vi "InitSupervisorCluster.vi"(8 "error in (no error)":errorcluster, 11 "ClusterIn in":T1={"Admin"={"Lvl"=enum."Admin", "Pwd"=""}, "RTConfig"={"Arm"=FALSE, "Number"=0.0, "String"=""}, "SMS"={"Enbl?"=FALSE, "Addr"=[]}, "FPGA"={"Target"=enum."1", "Channel"=enum."1", "Ref1"=refnum, "Ref2"=refnum}, "Config"={"UsrCfg"={"Paths"={"CfgFile"=path "", "LogFolder"=path "", "LogFile"=path "", "NAS path"=path "", "ThreshFile"=path "", "RedunFolder"=path ""}, "SampleRate"=0.0}, "FP_User"={"#NoiseSums"=0, "Max_df"=0, "AvgAvg"=FALSE, "#Avg"=0, "AutoCenter"=FALSE, "Inclin"={"Vmin"=0.0, "Vmax"=0.0, "Angle_min"=0.0, "Angle_max"=0.0, "Offset"=0.0, "Pos_Neg"=FALSE}, "1"={"Cal_"={"Fine"=0.0, "Coarse_"=0.0}, "Beac"={"Fine"=0.0, "Coarse_"=0.0}, "Scale"={"Step4"=0.0, "Step5"=0.0, "Step6"=0.0, "Step7"=0.0}, "Offset"=0.0, "Scale_Noise"=0.0, "Scale_Step1"=0.0, "Scale_In_RT"=0.0, "ScaleMeas"=0.0, "FreqsToRemove"=[], "Width"=[], "ScaleMeasEnum"=enum."1", "FilterEnab"=enum."None"}, "2"={"Cal_"={"Fine"=0.0, "Coarse_"=0.0}, "Beac"={"Fine"=0.0, "Coarse_"=0.0}, "Scale"={"Step4"=0.0, "Step5"=0.0, "Step6"=0.0, "Step7"=0.0}, "Offset"=0.0, "Scale_Noise"=0.0, "Scale_Step1"=0.0, "Scale_In_RT"=0.0, "ScaleMeas"=0.0, "FreqsToRemove"=[], "Width"=[], "ScaleMeasEnum"=enum."1", "FilterEnab"=enum."None"}, "3"={"Cal_"={"Fine"=0.0, "Coarse_"=0.0}, "Beac"={"Fine"=0.0, "Coarse_"=0.0}, "Scale"={"Step4"=0.0, "Step5"=0.0, "Step6"=0.0, "Step7"=0.0}, "Offset"=0.0, "Scale_Noise"=0.0, "Scale_Step1"=0.0, "Scale_In_RT"=0.0, "ScaleMeas"=0.0, "FreqsToRemove"=[], "Width"=[], "ScaleMeasEnum"=enum."1", "FilterEnab"=enum."None"}, "4"={"Cal_"={"Fine"=0.0, "Coarse_"=0.0}, "Beac"={"Fine"=0.0, "Coarse_"=0.0}, "Scale"={"Step4"=0.0, "Step5"=0.0, "Step6"=0.0, "Step7"=0.0}, "Offset"=0.0, "Scale_Noise"=0.0, "Scale_Step1"=0.0, "Scale_In_RT"=0.0, "ScaleMeas"=0.0, "FreqsToRemove"=[], "Width"=[], "ScaleMeasEnum"=enum."1", "FilterEnab"=enum."None"}, "Target to Probe"=enum."1", "SNR_Thresh"=0.0, "Paths"={"CfgFile"=path "", "LogFolder"=path "", "LogFile"=path "", "NAS path"=path "", "ThreshFile"=path "", "RedunFolder"=path ""}, "Connex_Location"="", "SimulateFPGA"=FALSE, "Deadband"=0.0}}, "Stat"={"SysState"=enum."Init", "TrackRate"=FALSE, "AutoCentr"=FALSE}, "Alarm"={"TC13"={"Enbl"=FALSE, "ErrsAndWarns"={0.0, 5.663716814159292, 7.168141592920354, 8.584070796460177}}, "AI1"={"Enbl"=FALSE, "ErrsAndWarns"={0.0, 5.663716814159292, 7.168141592920354, 8.584070796460177}}, "AI2"={"Enbl"=FALSE, "ErrsAndWarns"={0.0, 5.663716814159292, 7.168141592920354, 8.584070796460177}}, "AI3"={"Enbl"=FALSE, "ErrsAndWarns"={0.0, 5.663716814159292, 7.168141592920354, 8.584070796460177}}, "AI4"={"Enbl"=FALSE, "ErrsAndWarns"={0.0, 5.663716814159292, 7.168141592920354, 8.584070796460177}}, "AI5"={"Enbl"=FALSE, "ErrsAndWarns"={0.0, 5.663716814159292, 7.168141592920354, 8.584070796460177}}, "AI6"={"Enbl"=FALSE, "ErrsAndWarns"={0.0, 5.663716814159292, 7.168141592920354, 8.584070796460177}}, "AI18"={"Enbl"=FALSE, "ErrsAndWarns"={0.0, 5.663716814159292, 7.168141592920354, 8.584070796460177}}, "AI19"={"Enbl"=FALSE, "ErrsAndWarns"={0.0, 5.663716814159292, 7.168141592920354, 8.584070796460177}}, "TE1"={"Enbl"=FALSE, "ErrsAndWarns"={0.0, 5.663716814159292, 7.168141592920354, 8.584070796460177}}, "TE2"={"Enbl"=TRUE, "ErrsAndWarns"={0.0, 5.663716814159292, 7.168141592920354, 8.584070796460177}}, "TE3"={"Enbl"=FALSE, "ErrsAndWarns"={0.0, 5.663716814159292, 7.168141592920354, 8.584070796460177}}, "ADAM1"={"Enbl"=FALSE, "ErrsAndWarns"={0.0, 5.663716814159292, 7.168141592920354, 8.584070796460177}}, "ADAM2"={"Enbl"=FALSE, "ErrsAndWarns"={0.0, 5.663716814159292, 7.168141592920354, 8.584070796460177}}, "ADAM3"={"Enbl"=FALSE, "ErrsAndWarns"={0.0, 5.663716814159292, 7.168141592920354, 8.584070796460177}}, "ADAM4"={"Enbl"=FALSE, "ErrsAndWarns"={0.0, 5.663716814159292, 7.168141592920354, 8.584070796460177}}, "72CoBeacFreq"={"Enbl"=FALSE, "ErrsAndWarns"={0.0, 5.663716814159292, 7.168141592920354, 8.584070796460177}}, "72CoCalFreq"={"Enbl"=FALSE, "ErrsAndWarns"={0.0, 5.663716814159292, 7.168141592920354, 8.584070796460177}}, "84CoBeacFreq"={"Enbl"=FALSE, "ErrsAndWarns"={0.0, 5.663716814159292, 7.168141592920354, 8.584070796460177}}, "84CoCalFreq"={"Enbl"=FALSE, "ErrsAndWarns"={0.0, 5.663716814159292, 7.168141592920354, 8.584070796460177}}, "72Co_CalTonePwr"={"Enbl"=FALSE, "ErrsAndWarns"={0.0, 5.663716814159292, 7.168141592920354, 8.584070796460177}}, "72X_CalTonePwr"={"Enbl"=FALSE, "ErrsAndWarns"={0.0, 5.663716814159292, 7.168141592920354, 8.584070796460177}}, "84Co_CalTonePwr"={"Enbl"=FALSE, "ErrsAndWarns"={0.0, 5.663716814159292, 7.168141592920354, 8.584070796460177}}, "84X_CalTonePwr"={"Enbl"=FALSE, "ErrsAndWarns"={0.0, 5.663716814159292, 7.168141592920354, 8.584070796460177}}}} {"Alarm"."84X_CalTonePwr"."ErrsAndWarns" scale=-120.0..-45.0; "Alarm"."72X_CalTonePwr"."ErrsAndWarns" scale=-120.0..-45.0; "Alarm"."84Co_CalTonePwr"."ErrsAndWarns" scale=-120.0..-45.0; "Alarm"."72Co_CalTonePwr"."ErrsAndWarns" scale=-120.0..-45.0; "Alarm"."84CoCalFreq"."ErrsAndWarns" scale=24.9..25.1; "Alarm"."84CoBeacFreq"."ErrsAndWarns" scale=25.5..27.0; "Alarm"."72CoCalFreq"."ErrsAndWarns" scale=24.9..25.1; "Alarm"."72CoBeacFreq"."ErrsAndWarns" scale=25.5..27.0; "Alarm"."ADAM4"."ErrsAndWarns" scale=30.0..52.0; "Alarm"."ADAM3"."ErrsAndWarns" scale=30.0..52.0; "Alarm"."ADAM2"."ErrsAndWarns" scale=30.0..52.0; "Alarm"."ADAM1"."ErrsAndWarns" scale=30.0..52.0; "Alarm"."TE3"."ErrsAndWarns" scale=30.0..52.0; "Alarm"."TE2"."ErrsAndWarns" scale=30.0..52.0; "Alarm"."TE1"."ErrsAndWarns" scale=20.0..52.0; "Alarm"."AI19"."ErrsAndWarns" scale=0.0..60.0; "Alarm"."AI18"."ErrsAndWarns" scale=-10.0..10.0; "Alarm"."AI6"."ErrsAndWarns" scale=0.0..35.0; "Alarm"."AI5"."ErrsAndWarns" scale=0.0..20.0; "Alarm"."AI4"."ErrsAndWarns" scale=0.0..15.0; "Alarm"."AI3"."ErrsAndWarns" scale=0.0..10.0; "Alarm"."AI2"."ErrsAndWarns" scale=0.0..10.0; "Alarm"."TC13"."ErrsAndWarns" scale=-10.0..40.0; "Config"."FP_User"."Deadband" format="%#.0f"}) -> (0 "error out":errorcluster, 3 "ClusterIn out":T1={"Admin"={"Lvl"=enum."Admin", "Pwd"=""}, "RTConfig"={"Arm"=FALSE, "Number"=0.0, "String"=""}, "SMS"={"Enbl?"=FALSE, "Addr"=[]}, "FPGA"={"Target"=enum."1", "Channel"=enum."1", "Ref1"=refnum, "Ref2"=refnum}, "Config"={"UsrCfg"={"Paths"={"CfgFile"=path "", "LogFolder"=path "", "LogFile"=path "", "NAS path"=path "", "ThreshFile"=path "", "RedunFolder"=path ""}, "SampleRate"=0.0}, "FP_User"={"#NoiseSums"=0, "Max_df"=0, "AvgAvg"=FALSE, "#Avg"=0, "AutoCenter"=FALSE, "Inclin"={"Vmin"=0.0, "Vmax"=0.0, "Angle_min"=0.0, "Angle_max"=0.0, "Offset"=0.0, "Pos_Neg"=FALSE}, "1"={"Cal_"={"Fine"=0.0, "Coarse_"=0.0}, "Beac"={"Fine"=0.0, "Coarse_"=0.0}, "Scale"={"Step4"=0.0, "Step5"=0.0, "Step6"=0.0, "Step7"=0.0}, "Offset"=0.0, "Scale_Noise"=0.0, "Scale_Step1"=0.0, "Scale_In_RT"=0.0, "ScaleMeas"=0.0, "FreqsToRemove"=[], "Width"=[], "ScaleMeasEnum"=enum."1", "FilterEnab"=enum."None"}, "2"={"Cal_"={"Fine"=0.0, "Coarse_"=0.0}, "Beac"={"Fine"=0.0, "Coarse_"=0.0}, "Scale"={"Step4"=0.0, "Step5"=0.0, "Step6"=0.0, "Step7"=0.0}, "Offset"=0.0, "Scale_Noise"=0.0, "Scale_Step1"=0.0, "Scale_In_RT"=0.0, "ScaleMeas"=0.0, "FreqsToRemove"=[], "Width"=[], "ScaleMeasEnum"=enum."1", "FilterEnab"=enum."None"}, "3"={"Cal_"={"Fine"=0.0, "Coarse_"=0.0}, "Beac"={"Fine"=0.0, "Coarse_"=0.0}, "Scale"={"Step4"=0.0, "Step5"=0.0, "Step6"=0.0, "Step7"=0.0}, "Offset"=0.0, "Scale_Noise"=0.0, "Scale_Step1"=0.0, "Scale_In_RT"=0.0, "ScaleMeas"=0.0, "FreqsToRemove"=[], "Width"=[], "ScaleMeasEnum"=enum."1", "FilterEnab"=enum."None"}, "4"={"Cal_"={"Fine"=0.0, "Coarse_"=0.0}, "Beac"={"Fine"=0.0, "Coarse_"=0.0}, "Scale"={"Step4"=0.0, "Step5"=0.0, "Step6"=0.0, "Step7"=0.0}, "Offset"=0.0, "Scale_Noise"=0.0, "Scale_Step1"=0.0, "Scale_In_RT"=0.0, "ScaleMeas"=0.0, "FreqsToRemove"=[], "Width"=[], "ScaleMeasEnum"=enum."1", "FilterEnab"=enum."None"}, "Target to Probe"=enum."1", "SNR_Thresh"=0.0, "Paths"={"CfgFile"=path "", "LogFolder"=path "", "LogFile"=path "", "NAS path"=path "", "ThreshFile"=path "", "RedunFolder"=path ""}, "Connex_Location"="", "SimulateFPGA"=FALSE, "Deadband"=0.0}}, "Stat"={"SysState"=enum."Init", "TrackRate"=FALSE, "AutoCentr"=FALSE}, "Alarm"={"TC13"={"Enbl"=FALSE, "ErrsAndWarns"={0.0, 5.663716814159292, 7.168141592920354, 8.584070796460177}}, "AI1"={"Enbl"=FALSE, "ErrsAndWarns"={0.0, 5.663716814159292, 7.168141592920354, 8.584070796460177}}, "AI2"={"Enbl"=FALSE, "ErrsAndWarns"={0.0, 5.663716814159292, 7.168141592920354, 8.584070796460177}}, "AI3"={"Enbl"=FALSE, "ErrsAndWarns"={0.0, 5.663716814159292, 7.168141592920354, 8.584070796460177}}, "AI4"={"Enbl"=FALSE, "ErrsAndWarns"={0.0, 5.663716814159292, 7.168141592920354, 8.584070796460177}}, "AI5"={"Enbl"=FALSE, "ErrsAndWarns"={0.0, 5.663716814159292, 7.168141592920354, 8.584070796460177}}, "AI6"={"Enbl"=FALSE, "ErrsAndWarns"={0.0, 5.663716814159292, 7.168141592920354, 8.584070796460177}}, "AI18"={"Enbl"=FALSE, "ErrsAndWarns"={0.0, 5.663716814159292, 7.168141592920354, 8.584070796460177}}, "AI19"={"Enbl"=FALSE, "ErrsAndWarns"={0.0, 5.663716814159292, 7.168141592920354, 8.584070796460177}}, "TE1"={"Enbl"=FALSE, "ErrsAndWarns"={0.0, 5.663716814159292, 7.168141592920354, 8.584070796460177}}, "TE2"={"Enbl"=TRUE, "ErrsAndWarns"={0.0, 5.663716814159292, 7.168141592920354, 8.584070796460177}}, "TE3"={"Enbl"=FALSE, "ErrsAndWarns"={0.0, 5.663716814159292, 7.168141592920354, 8.584070796460177}}, "ADAM1"={"Enbl"=FALSE, "ErrsAndWarns"={0.0, 5.663716814159292, 7.168141592920354, 8.584070796460177}}, "ADAM2"={"Enbl"=FALSE, "ErrsAndWarns"={0.0, 5.663716814159292, 7.168141592920354, 8.584070796460177}}, "ADAM3"={"Enbl"=FALSE, "ErrsAndWarns"={0.0, 5.663716814159292, 7.168141592920354, 8.584070796460177}}, "ADAM4"={"Enbl"=FALSE, "ErrsAndWarns"={0.0, 5.663716814159292, 7.168141592920354, 8.584070796460177}}, "72CoBeacFreq"={"Enbl"=FALSE, "ErrsAndWarns"={0.0, 5.663716814159292, 7.168141592920354, 8.584070796460177}}, "72CoCalFreq"={"Enbl"=FALSE, "ErrsAndWarns"={0.0, 5.663716814159292, 7.168141592920354, 8.584070796460177}}, "84CoBeacFreq"={"Enbl"=FALSE, "ErrsAndWarns"={0.0, 5.663716814159292, 7.168141592920354, 8.584070796460177}}, "84CoCalFreq"={"Enbl"=FALSE, "ErrsAndWarns"={0.0, 5.663716814159292, 7.168141592920354, 8.584070796460177}}, "72Co_CalTonePwr"={"Enbl"=FALSE, "ErrsAndWarns"={0.0, 5.663716814159292, 7.168141592920354, 8.584070796460177}}, "72X_CalTonePwr"={"Enbl"=FALSE, "ErrsAndWarns"={0.0, 5.663716814159292, 7.168141592920354, 8.584070796460177}}, "84Co_CalTonePwr"={"Enbl"=FALSE, "ErrsAndWarns"={0.0, 5.663716814159292, 7.168141592920354, 8.584070796460177}}, "84X_CalTonePwr"={"Enbl"=FALSE, "ErrsAndWarns"={0.0, 5.663716814159292, 7.168141592920354, 8.584070796460177}}}} {"Alarm"."84X_CalTonePwr"."ErrsAndWarns" scale=-120.0..-45.0; "Alarm"."72X_CalTonePwr"."ErrsAndWarns" scale=-120.0..-45.0; "Alarm"."84Co_CalTonePwr"."ErrsAndWarns" scale=-120.0..-45.0; "Alarm"."72Co_CalTonePwr"."ErrsAndWarns" scale=-120.0..-45.0; "Alarm"."84CoCalFreq"."ErrsAndWarns" scale=24.9..25.1; "Alarm"."84CoBeacFreq"."ErrsAndWarns" scale=25.5..27.0; "Alarm"."72CoCalFreq"."ErrsAndWarns" scale=24.9..25.1; "Alarm"."72CoBeacFreq"."ErrsAndWarns" scale=25.5..27.0; "Alarm"."ADAM4"."ErrsAndWarns" scale=30.0..52.0; "Alarm"."ADAM3"."ErrsAndWarns" scale=30.0..52.0; "Alarm"."ADAM2"."ErrsAndWarns" scale=30.0..52.0; "Alarm"."ADAM1"."ErrsAndWarns" scale=30.0..52.0; "Alarm"."TE3"."ErrsAndWarns" scale=30.0..52.0; "Alarm"."TE2"."ErrsAndWarns" scale=30.0..52.0; "Alarm"."TE1"."ErrsAndWarns" scale=20.0..52.0; "Alarm"."AI19"."ErrsAndWarns" scale=0.0..60.0; "Alarm"."AI18"."ErrsAndWarns" scale=-10.0..10.0; "Alarm"."AI6"."ErrsAndWarns" scale=0.0..35.0; "Alarm"."AI5"."ErrsAndWarns" scale=0.0..20.0; "Alarm"."AI4"."ErrsAndWarns" scale=0.0..15.0; "Alarm"."AI3"."ErrsAndWarns" scale=0.0..10.0; "Alarm"."AI2"."ErrsAndWarns" scale=0.0..10.0; "Alarm"."TC13"."ErrsAndWarns" scale=-10.0..40.0; "Config"."FP_User"."Deadband" format="%#.0f"})   [LabVIEW 2018]
uses:
  Controls/MasterCluster.ctl
  Controls/Clusts/AdminCluster.ctl
  Controls/UserLevelEnum.ctl
  Controls/RT_Config.ctl
  Controls/SMSDataCluster.ctl
  Controls/Clusts/FPGA_Config_Clust.ctl
  Controls/Enums/TargetNumber.ctl
  Controls/Clusts/Config_Clust.ctl
  Controls/Clusts/UserConfig.ctl
  Controls/PathsCluster.ctl
  Controls/Clusts/FrontPanel_UserConfig.ctl
  Controls/Clusts/Inclinometer_User_Cfg.ctl
  Controls/Clusts/FP_UserTargetConfig.ctl
  Controls/Clusts/FreqShift.ctl
  Controls/Clusts/FPGA_Scale.ctl
  Controls/Enums/ScaleMeasure.ctl
  Controls/RadioButtons/FilterEnableRadio.ctl
  Controls/SystemStatusCluster.ctl
  Controls/SystemStateEnum.ctl
  Controls/Clusts/AlarmSettingsClust.ctl
  Controls/Clusts/AlarmThresh_OneChan.ctl
  <vilib>/Utility/sysdir.llb/System Directory Type.ctl
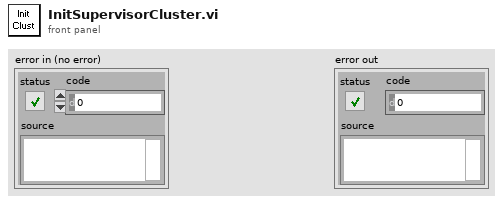
[diagram p1: front panel]
types:
  T1 = typedef "MasterCluster.ctl" = cluster{"Admin":T2, "RTConfig":T4, "SMS":T5, "FPGA":T6, "Config":T8, "Stat":T18, "Alarm":T20}
  T2 = typedef "AdminCluster.ctl" = cluster{"Lvl":T3, "Pwd":string}
  T3 = typedef "UserLevelEnum.ctl" = enum16{"Admin", "Operator"}
  T4 = typedef "RT_Config.ctl" = cluster{"Arm":bool, "Number":dbl, "String":string}
  T5 = typedef "SMSDataCluster.ctl" = cluster{"Enbl?":bool, "Addr":string[]}
  T6 = typedef "FPGA_Config_Clust.ctl" = cluster{"Target":T7, "Channel":T7, "Ref1":refnum<k20>, "Ref2":refnum<k20>}
  T7 = typedef "TargetNumber.ctl" = enum16{"1", "2", "3", "4"}
  T8 = typedef "Config_Clust.ctl" = cluster{"UsrCfg":T9, "FP_User":T11}
  T9 = typedef "UserConfig.ctl" = cluster{"Paths":T10, "SampleRate":dbl}
  T10 = typedef "PathsCluster.ctl" = cluster{"CfgFile":path, "LogFolder":path, "LogFile":path, "NAS path":path, "ThreshFile":path, "RedunFolder":path}
  T11 = typedef "FrontPanel_UserConfig.ctl" = cluster{"#NoiseSums":u32, "Max_df":u32, "AvgAvg":bool, "#Avg":u16, "AutoCenter":bool, "Inclin":T12, "1":T13, "2":T13, "3":T13, "4":T13, "Target to Probe":T7, "SNR_Thresh":dbl, "Paths":T10, "Connex_Location":string, "SimulateFPGA":bool, "Deadband":dbl}
  T12 = typedef "Inclinometer_User_Cfg.ctl" = cluster{"Vmin":dbl, "Vmax":dbl, "Angle_min":dbl, "Angle_max":dbl, "Offset":dbl, "Pos_Neg":bool}
  T13 = typedef "FP_UserTargetConfig.ctl" = cluster{"Cal_":T14, "Beac":T14, "Scale":T15, "Offset":fxp<+/-,16,16>, "Scale_Noise":fxp<+/-,30,30>, "Scale_Step1":fxp<+/-,17,17>, "Scale_In_RT":ext, "ScaleMeas":fxp<+/-,16,1>, "FreqsToRemove":i32[], "Width":i32[], "ScaleMeasEnum":T16, "FilterEnab":T17}
  T14 = typedef "FreqShift.ctl" = cluster{"Fine":dbl, "Coarse_":dbl}
  T15 = typedef "FPGA_Scale.ctl" = cluster{"Step4":fxp<+/-,23,23>, "Step5":fxp<+/-,23,23>, "Step6":fxp<+/-,23,23>, "Step7":fxp<+/-,23,23>}
  T16 = typedef "ScaleMeasure.ctl" = enum16{"1", "10", "50", "42"}
  T17 = typedef "FilterEnableRadio.ctl" = enum32{"None", "Step 1", "Frequency Shift", "Step 4", "Step 5", "Step 6", "Step 7"}
  T18 = typedef "SystemStatusCluster.ctl" = cluster{"SysState":T19, "TrackRate":bool, "AutoCentr":bool}
  T19 = typedef "SystemStateEnum.ctl" = enum16{"Init", "Idle", "Running", "System Fault", "System Error", "Exit"}
  T20 = typedef "AlarmSettingsClust.ctl" = cluster{"TC13":T21, "AI1":T21, "AI2":T21, "AI3":T21, "AI4":T21, "AI5":T21, "AI6":T21, "AI18":T21, "AI19":T21, "TE1":T21, "TE2":T21, "TE3":T21, "ADAM1":T21, "ADAM2":T21, "ADAM3":T21, "ADAM4":T21, "72CoBeacFreq":T21, "72CoCalFreq":T21, "84CoBeacFreq":T21, "84CoCalFreq":T21, "72Co_CalTonePwr":T21, "72X_CalTonePwr":T21, "84Co_CalTonePwr":T21, "84X_CalTonePwr":T21}
  T21 = typedef "AlarmThresh_OneChan.ctl" = cluster{"Enbl":bool, "ErrsAndWarns":cluster{dbl, dbl, dbl, dbl}}
  T22 = typedef "System Directory Type.ctl" = i32
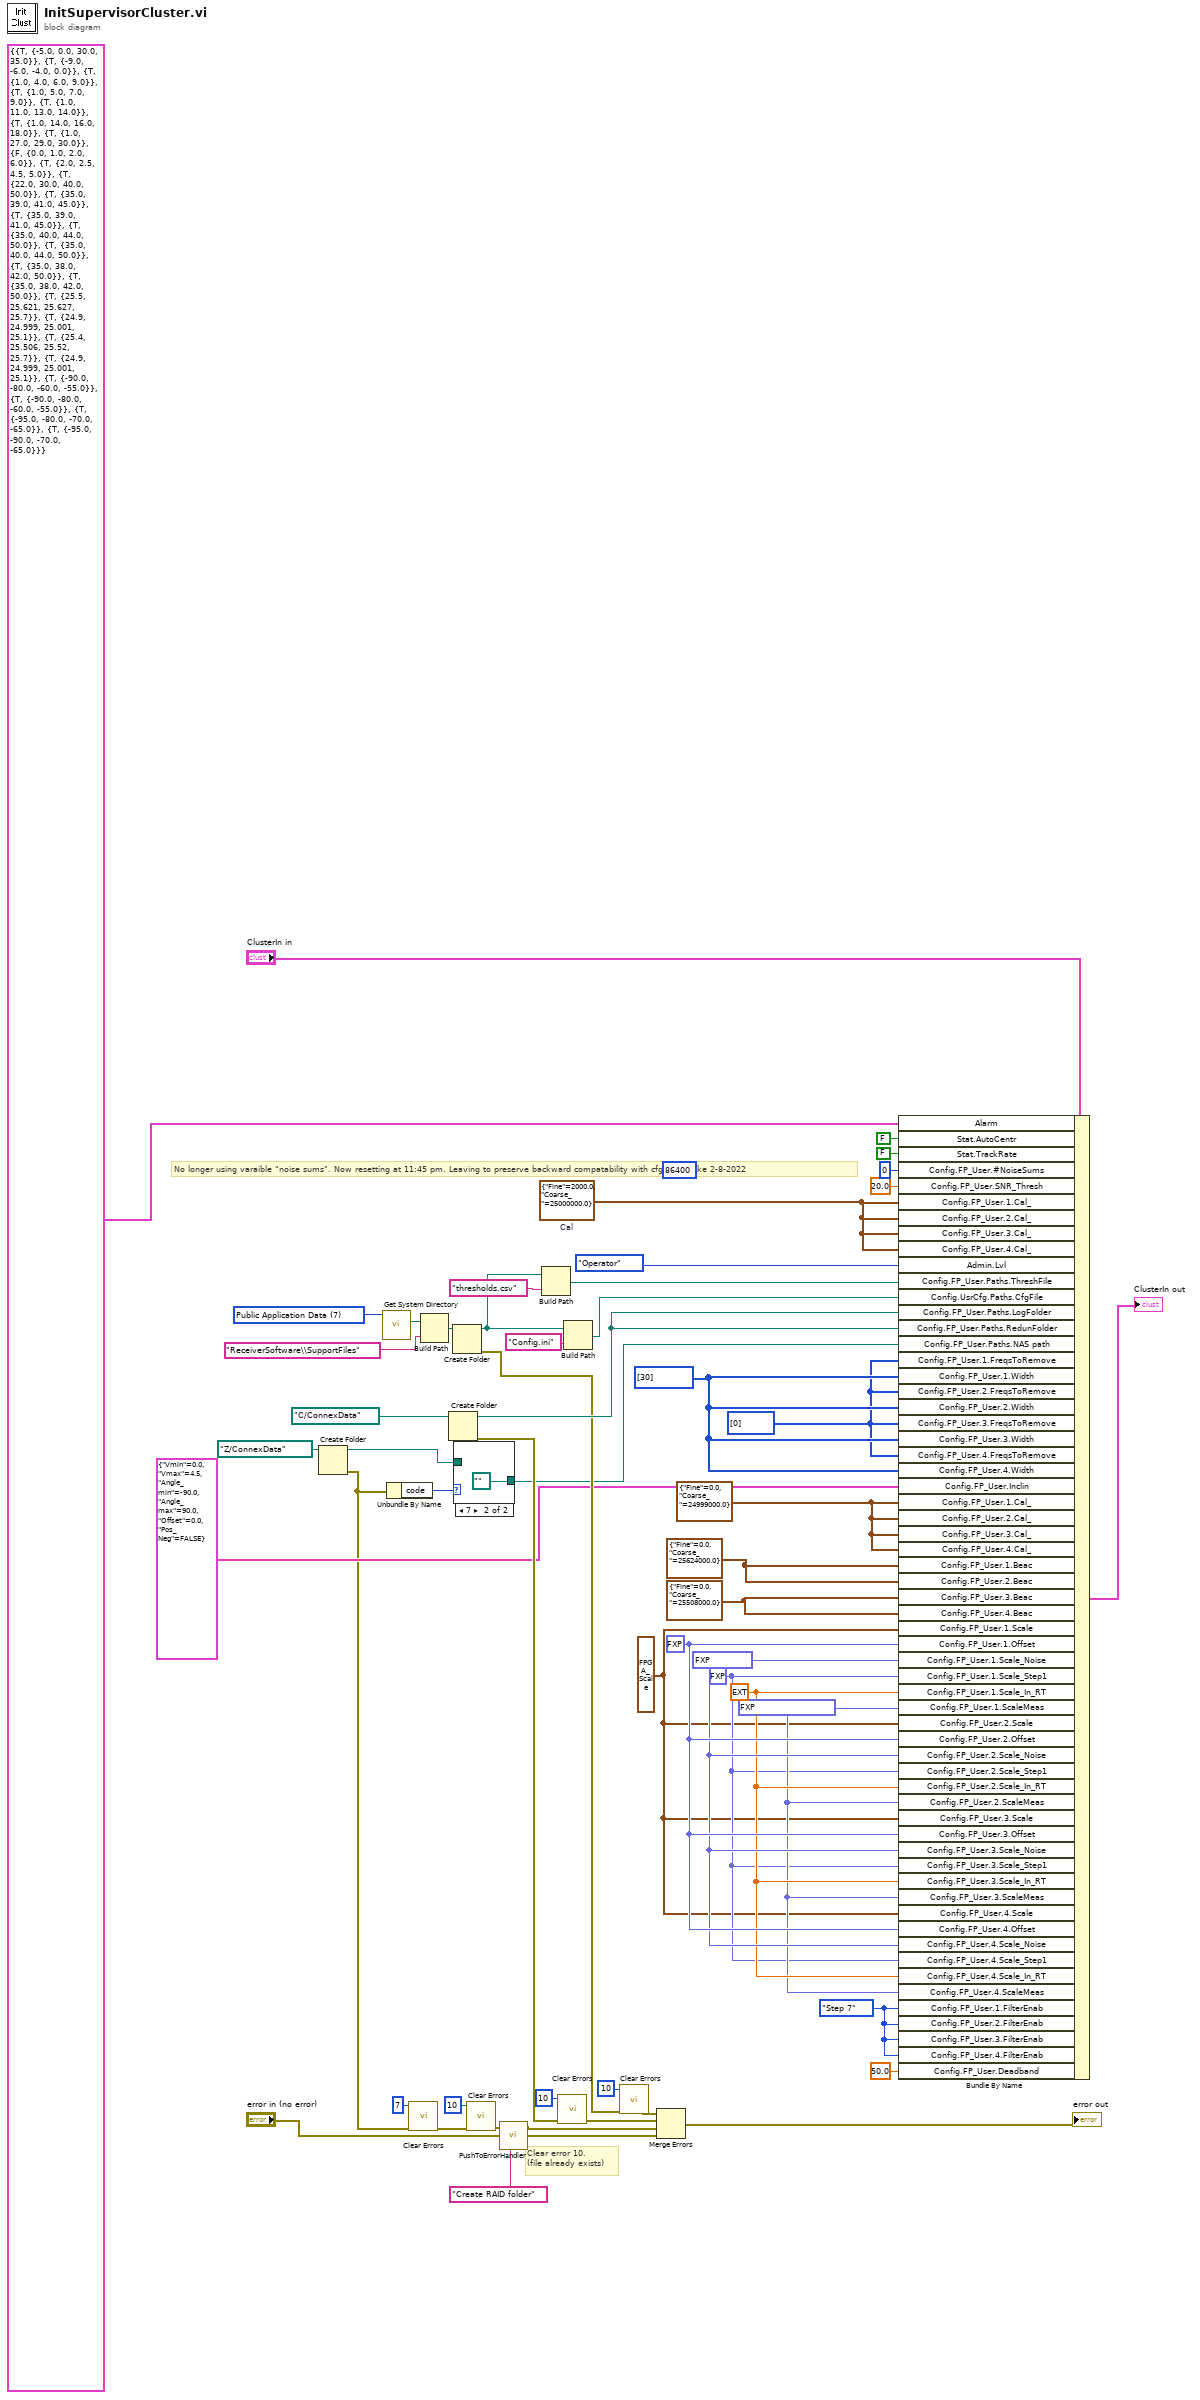
[diagram p0: block diagram]
diagram:
  w9 = FilterEnableRadio."Step 7" ("Config.FP_User.1.FilterEnab")
  w12 = fxp<+/-,16,1> 0.050018310546875 ("Config.FP_User.1.ScaleMeas")
  w13 = ext 1.0 ("Config.FP_User.1.Scale_In_RT")
  w14 = fxp<+/-,30,30> 536870911.0 ("Scale_NoiseFloor")
  w11 = fxp<+/-,17,17> 1.0 ("Config.FP_User.1.Scale_Step1")
  w15 = fxp<+/-,16,16> 0.0 ("Config.FP_User.1.Offset")
  w10 = T15 {"Step4"=3.0, "Step5"=1.0, "Step6"=1.0, "Step7"=1.0} ("Config.FP_User.1.Scale")
  w16 = T14 {"Fine"=0.0, "Coarse_"=25508000.0} ("Config.FP_User.1.Beac")
  w17 = T14 {"Fine"=0.0, "Coarse_"=25624000.0} ("Config.FP_User.1.Beac")
  w18 = T14 {"Fine"=0.0, "Coarse_"=24999000.0} ("Config.FP_User.1.Cal_")
  w52 = i32[] [30] ("Config.FP_User.4.Width")
  w51 = i32[] [0] ("Config.FP_User.1.FreqsToRemove")
  (unwired) u32 86400 ("Config.FP_User.#NoiseSums")
  w41 = T14 {"Fine"=2000.0, "Coarse_"=25000000.0}  # Cal
  w34 = T22 7 items=["User Home"=0, "User Desktop"=1, "User Documents"=2, "User Application Data"=3, "User Preferences"=4, "User Temporary"=5, "Public Documents"=6, "Public Application Data"=7, "Public Preferences"=8, "Public Cache"=13, "System Core Libraries"=9, "System Installed Libraries"=10, "Application Files"=11, "Boot Volume Root"=12] ("system directory type")
  # "No longer using varaible \"noise sums\". Now resetting at 11:45 pm. Leaving to preserve backward compatability with cfg files. Luke 2-8-2022"
  # "Clear error 10.\n(file already exists)"
  n1 = Create Folder(path (use dialog)=path "Z:/ConnexData" ("Config.FP_User.Paths.NAS path")) -> (created path=w6:path, error out=w4:errorcluster)  [unwired: 2 in, 1 out]
  n2 = call <vilib>:"Get System Directory.vi"("system directory type"=w34) -> ("system directory"=w36:path)  [unwired: 10 in]
  n3 = Unbundle By Name(w4) -> ("code"=w8:i32)
  n4 = call <vilib>:"Clear Errors.vi"("error in (no error)"=w4, "specific error code to clear (0: all)"=7) -> ("error out"=w3:errorcluster)  [unwired: 4 in, 1 out]
  n5 = Build Path(base path=w36, name or relative path="ReceiverSoftware\\SupportFiles") -> (appended path=w37:path)
  n6 = Create Folder(path (use dialog)=path "C:/ConnexData" ("Config.FP_User.Paths.LogFolder")) -> (created path=w47:path, error out=w27:errorcluster)  [unwired: 2 in, 1 out]
  n7 = Create Folder(path (use dialog)=w37) -> (created path=w23:path, error out=w30:errorcluster)  [unwired: 2 in, 1 out]
  n8 = case shown="7" w8 {
    tunnel: [w54 path "" ("created path")] -> w7
    tunnel: w6 -> [w54 _]
    frame Default {
    }
    frame 7 {
    }
  }
  n9 = call <vilib>:"Clear Errors.vi"("error in (no error)"=w3, "specific error code to clear (0: all)"=10) -> ("error out"=w21:errorcluster)  [unwired: 4 in, 1 out]
  n10 = call "PushToErrorHandler.vi"("ErrorIn"=w21, "ErrorLocation"="Create RAID folder") -> ("ErrorOut"=w22:errorcluster)  [unwired: 5 in]
  n11 = Build Path(base path=w23, name or relative path="thresholds.csv") -> (appended path=w46:path)
  n12 = call <vilib>:"Clear Errors.vi"("error in (no error)"=w27, "specific error code to clear (0: all)"=10) -> ("error out"=w28:errorcluster)  [unwired: 4 in, 1 out]
  n13 = Build Path(base path=w23, name or relative path="Config.ini") -> (appended path=w39:path)
  n14 = call <vilib>:"Clear Errors.vi"("error in (no error)"=w30, "specific error code to clear (0: all)"=10) -> ("error out"=w31:errorcluster)  [unwired: 4 in, 1 out]
  n15 = Merge Errors(w31, w28, w22, "error in (no error)") -> (→"error out":errorcluster)
  n16 = Bundle By Name(cluster="ClusterIn in", "Alarm"=T20 {"TC13"={"Enbl"=TRUE, "ErrsAndWarns"={-5.0, 0.0, 30.0, 35.0}}, "AI1"={"Enbl"=TRUE, "ErrsAndWarns"={-9.0, -6.0, -4.0, 0.0}}, "AI2"={"Enbl"=TRUE, "ErrsAndWarns"={1.0, 4.0, 6.0, 9.0}}, "AI3"={"Enbl"=TRUE, "ErrsAndWarns"={1.0, 5.0, 7.0, 9.0}}, "AI4"={"Enbl"=TRUE, "ErrsAndWarns"={1.0, 11.0, 13.0, 14.0}}, "AI5"={"Enbl"=TRUE, "ErrsAndWarns"={1.0, 14.0, 16.0, 18.0}}, "AI6"={"Enbl"=TRUE, "ErrsAndWarns"={1.0, 27.0, 29.0, 30.0}}, "AI18"={"Enbl"=FALSE, "ErrsAndWarns"={0.0, 1.0, 2.0, 6.0}}, "AI19"={"Enbl"=TRUE, "ErrsAndWarns"={2.0, 2.5, 4.5, 5.0}}, "TE1"={"Enbl"=TRUE, "ErrsAndWarns"={22.0, 30.0, 40.0, 50.0}}, "TE2"={"Enbl"=TRUE, "ErrsAndWarns"={35.0, 39.0, 41.0, 45.0}}, "TE3"={"Enbl"=TRUE, "ErrsAndWarns"={35.0, 39.0, 41.0, 45.0}}, "ADAM1"={"Enbl"=TRUE, "ErrsAndWarns"={35.0, 40.0, 44.0, 50.0}}, "ADAM2"={"Enbl"=TRUE, "ErrsAndWarns"={35.0, 40.0, 44.0, 50.0}}, "ADAM3"={"Enbl"=TRUE, "ErrsAndWarns"={35.0, 38.0, 42.0, 50.0}}, "ADAM4"={"Enbl"=TRUE, "ErrsAndWarns"={35.0, 38.0, 42.0, 50.0}}, "72CoBeacFreq"={"Enbl"=TRUE, "ErrsAndWarns"={25.5, 25.621, 25.627, 25.7}}, "72CoCalFreq"={"Enbl"=TRUE, "ErrsAndWarns"={24.9, 24.999, 25.001, 25.1}}, "84CoBeacFreq"={"Enbl"=TRUE, "ErrsAndWarns"={25.4, 25.506, 25.52, 25.7}}, "84CoCalFreq"={"Enbl"=TRUE, "ErrsAndWarns"={24.9, 24.999, 25.001, 25.1}}, "72Co_CalTonePwr"={"Enbl"=TRUE, "ErrsAndWarns"={-90.0, -80.0, -60.0, -55.0}}, "72X_CalTonePwr"={"Enbl"=TRUE, "ErrsAndWarns"={-90.0, -80.0, -60.0, -55.0}}, "84Co_CalTonePwr"={"Enbl"=TRUE, "ErrsAndWarns"={-95.0, -80.0, -70.0, -65.0}}, "84X_CalTonePwr"={"Enbl"=TRUE, "ErrsAndWarns"={-95.0, -90.0, -70.0, -65.0}}} ("AlarmSettings"), "Stat.AutoCentr"=FALSE, "Stat.TrackRate"=FALSE, "Config.FP_User.#NoiseSums"=u32 0, "Config.FP_User.SNR_Thresh"=20.0, "Config.FP_User.1.Cal_"=w41, "Config.FP_User.2.Cal_"=w41, "Config.FP_User.3.Cal_"=w41, "Config.FP_User.4.Cal_"=w41, "Admin.Lvl"=UserLevelEnum."Operator" ("User.Lvl"), "Config.FP_User.Paths.ThreshFile"=w46, "Config.UsrCfg.Paths.CfgFile"=w39, "Config.FP_User.Paths.LogFolder"=w47, "Config.FP_User.Paths.RedunFolder"=w47, "Config.FP_User.Paths.NAS path"=w7, "Config.FP_User.1.FreqsToRemove"=w51, "Config.FP_User.1.Width"=w52, "Config.FP_User.2.FreqsToRemove"=w51, "Config.FP_User.2.Width"=w52, "Config.FP_User.3.FreqsToRemove"=w51, "Config.FP_User.3.Width"=w52, "Config.FP_User.4.FreqsToRemove"=w51, "Config.FP_User.4.Width"=w52, "Config.FP_User.Inclin"=T12 {"Vmin"=0.0, "Vmax"=4.5, "Angle_min"=-90.0, "Angle_max"=90.0, "Offset"=0.0, "Pos_Neg"=FALSE}, "Config.FP_User.1.Cal_"=w18, "Config.FP_User.2.Cal_"=w18, "Config.FP_User.3.Cal_"=w18, "Config.FP_User.4.Cal_"=w18, "Config.FP_User.1.Beac"=w17, "Config.FP_User.2.Beac"=w17, "Config.FP_User.3.Beac"=w16, "Config.FP_User.4.Beac"=w16, "Config.FP_User.1.Scale"=w10, "Config.FP_User.1.Offset"=w15, "Config.FP_User.1.Scale_Noise"=w14, "Config.FP_User.1.Scale_Step1"=w11, "Config.FP_User.1.Scale_In_RT"=w13, "Config.FP_User.1.ScaleMeas"=w12, "Config.FP_User.2.Scale"=w10, "Config.FP_User.2.Offset"=w15, "Config.FP_User.2.Scale_Noise"=w14, "Config.FP_User.2.Scale_Step1"=w11, "Config.FP_User.2.Scale_In_RT"=w13, "Config.FP_User.2.ScaleMeas"=w12, "Config.FP_User.3.Scale"=w10, "Config.FP_User.3.Offset"=w15, "Config.FP_User.3.Scale_Noise"=w14, "Config.FP_User.3.Scale_Step1"=w11, "Config.FP_User.3.Scale_In_RT"=w13, "Config.FP_User.3.ScaleMeas"=w12, "Config.FP_User.4.Scale"=w10, "Config.FP_User.4.Offset"=w15, "Config.FP_User.4.Scale_Noise"=w14, "Config.FP_User.4.Scale_Step1"=w11, "Config.FP_User.4.Scale_In_RT"=w13, "Config.FP_User.4.ScaleMeas"=w12, "Config.FP_User.1.FilterEnab"=w9, "Config.FP_User.2.FilterEnab"=w9, "Config.FP_User.3.FilterEnab"=w9, "Config.FP_User.4.FilterEnab"=w9, "Config.FP_User.Deadband"=50.0) -> (→"ClusterIn out":T1)
